vi "CRYSet Acquisition Editor Front Panel.vi"(11 "Vi Ref":refnum<vi>) -> ()   [LabVIEW 2013]
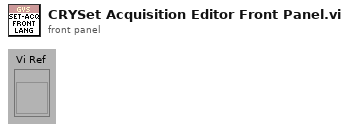
[diagram p1: front panel]
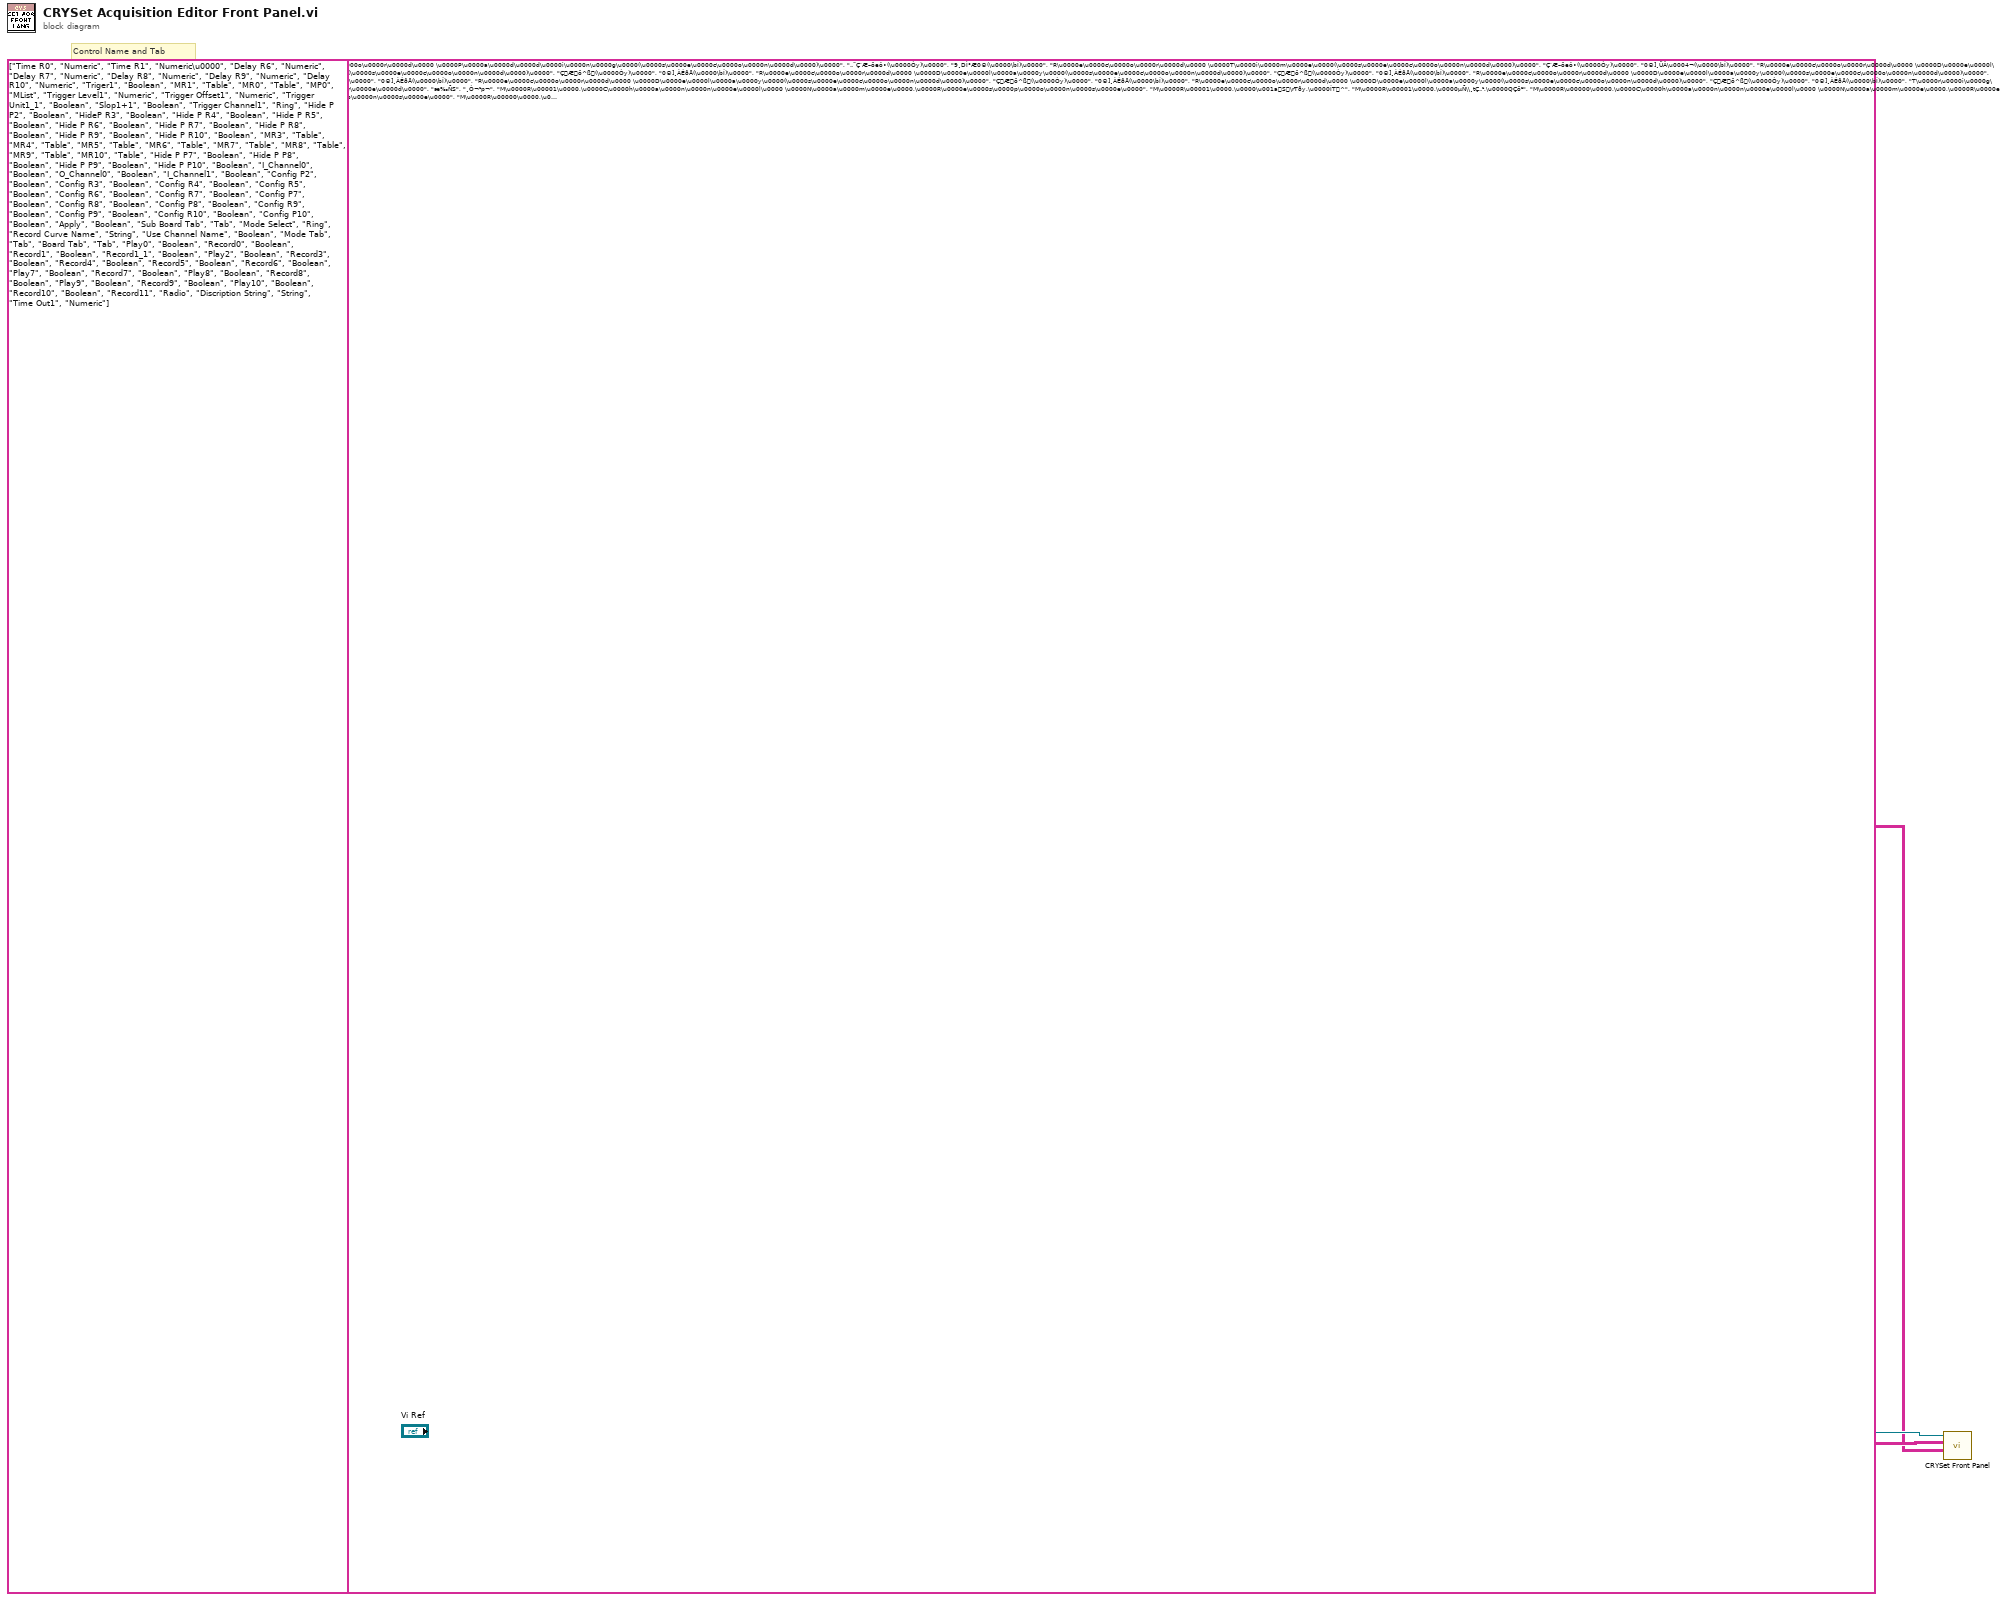
[diagram p0: block diagram]
diagram:
  # ","
  # "Caption, Tab Page, Multilist Header, Button 4"
  # "Control Type"
  # "Control Name and Tab"
  n1 = call "CRYSet Front Panel.vi"("Caption(Boolean Text)"=string[][] [["R\u0000e\u0000c\u0000o\u0000r\u0000d\u0000 \u0000P\u0000a\u0000d\u0000d\u0000i\u0000n\u0000g\u0000(\u0000s\u0000e\u0000c\u0000o\u0000n\u0000d\u0000)\u0000", "„˜Ç‘Æ–öeô•(\u0000Òy)\u0000", "9¸DÌ°Æ0®(\u0000\bÍ)\u0000"], ["R\u0000e\u0000c\u0000o\u0000r\u0000d\u0000 \u0000T\u0000i\u0000m\u0000e\u0000(\u0000s\u0000e\u0000c\u0000o\u0000n\u0000d\u0000)\u0000", "Ç‘Æ–öeô•(\u0000Òy)\u0000", "0®]¸ÜÂ\u0004¬(\u0000\bÍ)\u0000"], ["R\u0000e\u0000c\u0000o\u0000r\u0000d\u0000 \u0000D\u0000e\u0000l\u0000a\u0000y\u0000(\u0000s\u0000e\u0000c\u0000o\u0000n\u0000d\u0000)\u0000", "ÇÆö^ß(\u0000Òy)\u0000", "0®]¸ÀÉðÅ(\u0000\bÍ)\u0000"], ["R\u0000e\u0000c\u0000o\u0000r\u0000d\u0000 \u0000D\u0000e\u0000l\u0000a\u0000y\u0000(\u0000s\u0000e\u0000c\u0000o\u0000n\u0000d\u0000)\u0000", "ÇÆö^ß(\u0000Òy)\u0000", "0®]¸ÀÉðÅ(\u0000\bÍ)\u0000"], ["R\u0000e\u0000c\u0000o\u0000r\u0000d\u0000 \u0000D\u0000e\u0000l\u0000a\u0000y\u0000(\u0000s\u0000e\u0000c\u0000o\u0000n\u0000d\u0000)\u0000", "ÇÆö^ß(\u0000Òy)\u0000", "0®]¸ÀÉðÅ(\u0000\bÍ)\u0000"], ["R\u0000e\u0000c\u0000o\u0000r\u0000d\u0000 \u0000D\u0000e\u0000l\u0000a\u0000y\u0000(\u0000s\u0000e\u0000c\u0000o\u0000n\u0000d\u0000)\u0000", "ÇÆö^ß(\u0000Òy)\u0000", "0®]¸ÀÉðÅ(\u0000\bÍ)\u0000"], ["R\u0000e\u0000c\u0000o\u0000r\u0000d\u0000 \u0000D\u0000e\u0000l\u0000a\u0000y\u0000(\u0000s\u0000e\u0000c\u0000o\u0000n\u0000d\u0000)\u0000", "ÇÆö^ß(\u0000Òy)\u0000", "0®]¸ÀÉðÅ(\u0000\bÍ)\u0000"], ["T\u0000r\u0000i\u0000g\u0000g\u0000e\u0000r\u0000e\u0000d\u0000", "æ‰ÑS", "¸Ò¬¹p¬"], ["M\u0000R\u00001\u0000,\u0000C\u0000h\u0000a\u0000n\u0000n\u0000e\u0000l\u0000 \u0000N\u0000a\u0000m\u0000e\u0000,\u0000R\u0000e\u0000s\u0000p\u0000o\u0000n\u0000s\u0000e\u0000", "M\u0000R\u00001\u0000,\u0000\u001aS\rTðy,\u0000ÍT^", "M\u0000R\u00001\u0000,\u0000µÑ\\¸tÇ„¹,\u0000QÇõ²"], ["M\u0000R\u00000\u0000,\u0000C\u0000h\u0000a\u0000n\u0000n\u0000e\u0000l\u0000 \u0000N\u0000a\u0000m\u0000e\u0000,\u0000R\u0000e\u0000s\u0000p\u0000o\u0000n\u0000s\u0000e\u0000", "M\u0000R\u00000\u0000,\u0000\u001aS\rTðy,\u0000ÍT^", "M\u0000R\u00000\u0000,\u0000µÑ\\¸tÇ„¹,\u0000QÇõ²"], ["M\u0000P\u00000\u0000,\u0000C\u0000h\u0000a\u0000n\u0000n\u0000e\u0000l\u0000 \u0000N\u0000a\u0000m\u0000e\u0000,\u0000S\u0000t\u0000i\u0000m\u0000u\u0000l\u0000u\u0000s\u0000", "M\u0000P\u00000\u0000,\u0000\u001aS\rTðy,\u0000Ào±R", "M\u0000P\u0000,\u0000µÑ\\¸tÇ¹,\u0000Çù­"], ["T\u0000r\u0000i\u0000g\u0000g\u0000e\u0000r\u0000 \u0000L\u0000e\u0000v\u0000e\u0000l\u0000", "æ‰ÑS5us^", "¸Ò¬¹p¬\u0000É\u0004Ç"], ["T\u0000r\u0000i\u0000g\u0000g\u0000e\u0000r\u0000 \u0000O\u0000f\u0000f\u0000s\u0000e\u0000t\u0000(\u0000s\u0000)\u0000", "æ‰ÑSOPûy(\u0000s\u0000)\u0000", "¸Ò¬¹p¬¸Ó\u0004Ç(\u0000\bÍ)\u0000"], ["T\u0000r\u0000i\u0000g\u0000g\u0000e\u0000r\u0000 \u0000U\u0000n\u0000i\u0000t\u0000", "æ‰ÑSUSMO", "¸Ò¬¹p¬è²\u0004Ç"], ["S\u0000l\u0000o\u0000p\u0000e\u0000", "œe‡s", "½¬¬ÀÄ³"], ["T\u0000r\u0000i\u0000g\u0000g\u0000e\u0000r\u0000 \u0000C\u0000h\u0000a\u0000n\u0000n\u0000e\u0000l\u0000", "æÑS\u001aS", "¸Ò¬¹p¬µÑ\\¸"], ["H\u0000i\u0000d\u0000e\u0000 \u0000P\u0000a\u0000n\u0000e\u0000l\u0000", "Ïbg", "=Ì8»(Â0®0®"], ["H\u0000i\u0000d\u0000e\u0000 \u0000P\u0000a\u0000n\u0000e\u0000l\u0000", "Ïbg", "=Ì8»(Â0®0®"], ["H\u0000i\u0000d\u0000e\u0000 \u0000P\u0000a\u0000n\u0000e\u0000l\u0000", "Ïbg", "=Ì8»(Â0®0®"], ["H\u0000i\u0000d\u0000e\u0000 \u0000P\u0000a\u0000n\u0000e\u0000l\u0000", "Ïbg", "=Ì8»(Â0®0®"], ["H\u0000i\u0000d\u0000e\u0000 \u0000P\u0000a\u0000n\u0000e\u0000l\u0000", "Ïbg", "=Ì8»(Â0®0®"], ["H\u0000i\u0000d\u0000e\u0000 \u0000P\u0000a\u0000n\u0000e\u0000l\u0000", "Ïbg", "=Ì8»(Â0®0®"], ["H\u0000i\u0000d\u0000e\u0000 \u0000P\u0000a\u0000n\u0000e\u0000l\u0000", "Ïbg", "=Ì8»(Â0®0®"], ["H\u0000i\u0000d\u0000e\u0000 \u0000P\u0000a\u0000n\u0000e\u0000l\u0000", "Ïbg", "=Ì8»(Â0®0®"], ["H\u0000i\u0000d\u0000e\u0000 \u0000P\u0000a\u0000n\u0000e\u0000l\u0000", "Ïbg", "=Ì8»(Â0®0®"], ["M\u0000R\u00003\u0000,\u0000C\u0000h\u0000a\u0000n\u0000n\u0000e\u0000l\u0000 \u0000N\u0000a\u0000m\u0000e\u0000,\u0000R\u0000e\u0000s\u0000p\u0000o\u0000n\u0000s\u0000e\u0000", "M\u0000R\u00003\u0000,\u0000\u001aS\rTðy,\u0000ÍT^", "M\u0000R\u0000,\u0000µÑ\\¸tÇ„¹,\u0000QÇõ²"], ["M\u0000R\u00004\u0000,\u0000C\u0000h\u0000a\u0000n\u0000n\u0000e\u0000l\u0000 \u0000N\u0000a\u0000m\u0000e\u0000,\u0000R\u0000e\u0000s\u0000p\u0000o\u0000n\u0000s\u0000e\u0000", "M\u0000R\u00004\u0000,\u0000\u001aS\rTðy,\u0000ÍT^", "M\u0000R\u0000,\u0000µÑ\\¸tÇ„¹,\u0000QÇõ²"], ["M\u0000R\u00005\u0000,\u0000C\u0000h\u0000a\u0000n\u0000n\u0000e\u0000l\u0000 \u0000N\u0000a\u0000m\u0000e\u0000,\u0000R\u0000e\u0000s\u0000p\u0000o\u0000n\u0000s\u0000e\u0000", "M\u0000R\u00005\u0000,\u0000\u001aS\rTðy,\u0000ÍT^", "M\u0000R\u0000,\u0000µÑ\\¸tÇ„¹,\u0000QÇõ²"], ["M\u0000R\u00006\u0000,\u0000C\u0000h\u0000a\u0000n\u0000n\u0000e\u0000l\u0000 \u0000N\u0000a\u0000m\u0000e\u0000,\u0000R\u0000e\u0000s\u0000p\u0000o\u0000n\u0000s\u0000e\u0000", "M\u0000R\u00006\u0000,\u0000\u001aS\rTðy,\u0000ÍT^", "M\u0000R\u0000,\u0000µÑ\\¸tÇ„¹,\u0000QÇõ²"], ["M\u0000R\u00007\u0000,\u0000C\u0000h\u0000a\u0000n\u0000n\u0000e\u0000l\u0000 \u0000N\u0000a\u0000m\u0000e\u0000,\u0000R\u0000e\u0000s\u0000p\u0000o\u0000n\u0000s\u0000e\u0000", "M\u0000R\u00007\u0000,\u0000\u001aS\rTðy,\u0000ÍT^", "M\u0000R\u0000,\u0000µÑ\\¸tÇ„¹,\u0000QÇõ²"], ["M\u0000R\u00008\u0000,\u0000C\u0000h\u0000a\u0000n\u0000n\u0000e\u0000l\u0000 \u0000N\u0000a\u0000m\u0000e\u0000,\u0000R\u0000e\u0000s\u0000p\u0000o\u0000n\u0000s\u0000e\u0000", "M\u0000R\u00008\u0000,\u0000\u001aS\rTðy,\u0000ÍT^", "M\u0000R\u0000,\u0000µÑ\\¸tÇ„¹,\u0000QÇõ²"], ["M\u0000R\u00009\u0000,\u0000C\u0000h\u0000a\u0000n\u0000n\u0000e\u0000l\u0000 \u0000N\u0000a\u0000m\u0000e\u0000,\u0000R\u0000e\u0000s\u0000p\u0000o\u0000n\u0000s\u0000e\u0000", "M\u0000R\u00009\u0000,\u0000\u001aS\rTðy,\u0000ÍT^", "M\u0000R\u0000,\u0000µÑ\\¸tÇ„¹,\u0000QÇõ²"], ["M\u0000R\u00001\u00000\u0000,\u0000C\u0000h\u0000a\u0000n\u0000n\u0000e\u0000l\u0000 \u0000N\u0000a\u0000m\u0000e\u0000,\u0000R\u0000e\u0000s\u0000p\u0000o\u0000n\u0000s\u0000e\u0000", "M\u0000R\u00001\u00000\u0000,\u0000\u001aS\rTðy,\u0000ÍT^", "M\u0000R\u0000,\u0000µÑ\\¸tÇ„¹,\u0000QÇõ²"], ["H\u0000i\u0000d\u0000e\u0000 \u0000P\u0000a\u0000n\u0000e\u0000l\u0000", "Ïbg", "=Ì8»(Â0®0®"], ["H\u0000i\u0000d\u0000e\u0000 \u0000P\u0000a\u0000n\u0000e\u0000l\u0000", "Ïbg", "=Ì8»(Â0®0®"], ["H\u0000i\u0000d\u0000e\u0000 \u0000P\u0000a\u0000n\u0000e\u0000l\u0000", "Ïbg", "=Ì8»(Â0®0®"], ["H\u0000i\u0000d\u0000e\u0000 \u0000P\u0000a\u0000n\u0000e\u0000l\u0000", "Ïbg", "=Ì8»(Â0®0®"], ["I\u0000n\u0000p\u0000u\u0000t\u0000 \u0000C\u0000h\u0000a\u0000n\u0000n\u0000e\u0000l\u0000", "eQ\u001aS", "…Çl­µÑ\\¸"], ["O\u0000u\u0000t\u0000p\u0000u\u0000t\u0000 \u0000C\u0000h\u0000a\u0000n\u0000n\u0000e\u0000l\u0000", "úQ\u001aS", "œÍl­µÑ\\¸"], ["I\u0000n\u0000p\u0000u\u0000t\u0000 \u0000C\u0000h\u0000a\u0000n\u0000n\u0000e\u0000l\u0000", "eQ\u001aS", "…Çl­µÑ\\¸"], ["C\u0000o\u0000n\u0000f\u0000i\u0000g\u0000u\u0000r\u0000e\u0000 \u0000G\u0000e\u0000n\u0000e\u0000r\u0000a\u0000t\u0000o\u0000r\u0000", "M‘nÑS\u001fuhV", "\u001c¼ÝÀ0®l­1Á"], ["C\u0000o\u0000n\u0000f\u0000i\u0000g\u0000u\u0000r\u0000e\u0000 \u0000R\u0000e\u0000c\u0000o\u0000r\u0000d\u0000", "M‘n°‹U_", "0®]¸l­1Á"], ["C\u0000o\u0000n\u0000f\u0000i\u0000g\u0000u\u0000r\u0000e\u0000 \u0000R\u0000e\u0000c\u0000o\u0000r\u0000d\u0000", "M‘n°‹U_", "0®]¸l­1Á"], ["C\u0000o\u0000n\u0000f\u0000i\u0000g\u0000u\u0000r\u0000e\u0000 \u0000R\u0000e\u0000c\u0000o\u0000r\u0000d\u0000", "M‘n°‹U_", "0®]¸l­1Á"], ["C\u0000o\u0000n\u0000f\u0000i\u0000g\u0000u\u0000r\u0000e\u0000 \u0000R\u0000e\u0000c\u0000o\u0000r\u0000d\u0000", "M‘n°‹U_", "0®]¸l­1Á"], ["C\u0000o\u0000n\u0000f\u0000i\u0000g\u0000u\u0000r\u0000e\u0000 \u0000R\u0000e\u0000c\u0000o\u0000r\u0000d\u0000", "M‘n°‹U_", "0®]¸l­1Á"], ["C\u0000o\u0000n\u0000f\u0000i\u0000g\u0000u\u0000r\u0000e\u0000 \u0000G\u0000e\u0000n\u0000e\u0000r\u0000a\u0000t\u0000o\u0000r\u0000", "M‘nÑS\u001fuhV", "\u001c¼ÝÀ0®l­1Á"], ["C\u0000o\u0000n\u0000f\u0000i\u0000g\u0000u\u0000r\u0000e\u0000 \u0000R\u0000e\u0000c\u0000o\u0000r\u0000d\u0000", "M‘n°‹U_", "0®]¸l­1Á"], ["C\u0000o\u0000n\u0000f\u0000i\u0000g\u0000u\u0000r\u0000e\u0000 \u0000G\u0000e\u0000n\u0000e\u0000r\u0000a\u0000t\u0000o\u0000r\u0000", "M‘nÑS\u001fuhV", "\u001c¼ÝÀ0®l­1Á"], ["C\u0000o\u0000n\u0000f\u0000i\u0000g\u0000u\u0000r\u0000e\u0000 \u0000R\u0000e\u0000c\u0000o\u0000r\u0000d\u0000", "M‘n°‹U_", "0®]¸l­1Á"], ["C\u0000o\u0000n\u0000f\u0000i\u0000g\u0000u\u0000r\u0000e\u0000 \u0000G\u0000e\u0000n\u0000e\u0000r\u0000a\u0000t\u0000o\u0000r\u0000", "M‘nÑS\u001fuhV", "\u001c¼ÝÀ0®l­1Á"], ["C\u0000o\u0000n\u0000f\u0000i\u0000g\u0000u\u0000r\u0000e\u0000 \u0000R\u0000e\u0000c\u0000o\u0000r\u0000d\u0000", "M‘n°‹U_", "0®]¸l­1Á"], ["C\u0000o\u0000n\u0000f\u0000i\u0000g\u0000u\u0000r\u0000e\u0000 \u0000G\u0000e\u0000n\u0000e\u0000r\u0000a\u0000t\u0000o\u0000r\u0000", "M‘nÑS\u001fuhV", "\u001c¼ÝÀ0®l­1Á"], ["A\u0000p\u0000p\u0000l\u0000y\u0000,\u0000S\u0000t\u0000o\u0000p\u0000", "”^(u,\u0000\\Pbk", "\u0001È©Æ,\u0000\u0015ÈÀÉ"], ["S\u0000e\u0000t\u0000t\u0000i\u0000n\u0000g\u0000,\u0000H\u0000e\u0000l\u0000p\u0000", "¾‹n,\u0000.^©R", "$Á\u0015È,\u0000Ä³ÀÆÐ¹"], ["M\u0000o\u0000d\u0000e\u0000 \u0000S\u0000e\u0000l\u0000e\u0000c\u0000t\u0000,\u0000P\u0000l\u0000a\u0000y\u0000 \u0000&\u0000 \u0000R\u0000e\u0000c\u0000o\u0000r\u0000d\u0000,\u0000R\u0000e\u0000c\u0000o\u0000r\u0000d\u0000,\u0000S\u0000i\u0000g\u0000n\u0000a\u0000l\u0000 \u0000G\u0000e\u0000n\u0000e\u0000r\u0000a\u0000t\u0000o\u0000r\u0000,\u0000M\u0000u\u0000l\u0000t\u0000i\u0000m\u0000e\u0000t\u0000e\u0000r\u0000,\u0000O\u0000s\u0000c\u0000i\u0000l\u0000l\u0000o\u0000s\u0000c\u0000o\u0000p\u0000e\u0000,\u0000S\u0000p\u0000e\u0000c\u0000t\u0000r\u0000u\u0000m\u0000 \u0000A\u0000n\u0000a\u0000l\u0000y\u0000z\u0000e\u0000r\u0000,\u0000R\u0000e\u0000a\u0000l\u0000 \u0000T\u0000i\u0000m\u0000e\u0000 \u0000A\u0000n\u0000a\u0000l\u0000y\u0000z\u0000e\u0000r\u0000,\u0000G\u0000e\u0000n\u0000e\u0000r\u0000a\u0000t\u0000o\u0000r\u0000 \u0000&\u0000 \u0000M\u0000u\u0000l\u0000t\u0000i\u0000m\u0000e\u0000t\u0000e\u0000r\u0000,\u0000G\u0000e\u0000n\u0000e\u0000r\u0000a\u0000t\u0000o\u0000r\u0000 \u0000&\u0000 \u0000O\u0000s\u0000c\u0000i\u0000l\u0000l\u0000o\u0000s\u0000c\u0000o\u0000p\u0000e\u0000,\u0000G\u0000e\u0000n\u0000e\u0000r\u0000a\u0000t\u0000o\u0000r\u0000 \u0000&\u0000 \u0000S\u0000p\u0000e\u0000c\u0000t\u0000r\u0000u\u0000m\u0000,\u0000G\u0000e\u0000n\u0000e\u0000r\u0000a\u0000t\u0000o\u0000r\u0000 \u0000&\u0000 \u0000R\u0000T\u0000A\u0000,\u0000R\u0000e\u0000a\u0000d\u0000 \u0000f\u0000r\u0000o\u0000m\u0000 \u0000D\u0000C\u0000 \u0000C\u0000o\u0000n\u0000n\u0000e\u0000c\u0000t\u0000", "!j\u000f_\téb,\u0000­d>eTÇÆ,\u0000ÇÆ,\u0000áO÷SÑS\u001fuhV,\u0000\u001aYRýh,\u0000:yâlhV,\u00001\u0006RgêN,\u0000[öe1\u0006RgêN,\u0000áO÷SÑS\u001fuhV/\u0000\u001aYRýh,\u0000áO÷SÑS\u001fuhV/\u0000:yâlhV,\u0000áO÷SÑS\u001fuhV/\u00001\u0006RgêN,\u0000áO÷SÑS\u001fuhV/\u0000[öe1\u0006RgêN,\u0000ûÖSôvAmÞ¥c", ")¼ÝÂ ÁÝÐ,\u0000¬ÇÝÀü¬ \u00000®]¸,\u00000®]¸,\u0000àÂ8Ö\u001c¼ÝÀ0®,\u0000Ì¹¥²!Î\u0015ÈÄ¬0®,\u0000$Æ0Å\\¸¤ÂTÏ\u0004Õ,\u0000¤Â™Ó¸Òt¹„½\u001dÁ0®,\u0000%ÆÀÐ\f¾„½\u001dÁ0®,\u0000àÂ8Ö\u001c¼ÝÀ0®@Æ \u0000Ì¹¥²!Î\u0015ÈÄ¬0®,\u0000àÂ8Ö\u001c¼ÝÀ0®@Æ \u0000$Æ0Å\\¸¤ÂTÏ\u0004Õ,\u0000àÂ8Ö\u001c¼ÝÀ0®@Æ \u0000¤Â™Ó¸Òt¹„½\u001dÁ0®,\u0000àÂ8Ö\u001c¼ÝÀ0®@Æ \u0000%ÆÀÐ\f¾„½\u001dÁ0®,\u0000ÁÉX¹(¸°¬0®\\¸ \u0000€½0Ñ \u0000}Ç0®"], ["R\u0000e\u0000c\u0000o\u0000r\u0000d\u0000 \u0000C\u0000u\u0000r\u0000v\u0000e\u0000 \u0000N\u0000a\u0000m\u0000e\u0000", "°‹U_òf¿~\rTðy", "0®]¸á¬ ÁtÇ„¹"], ["U\u0000s\u0000e\u0000 \u0000C\u0000h\u0000a\u0000n\u0000n\u0000e\u0000l\u0000 \u0000N\u0000a\u0000m\u0000e\u0000", "O(u\u001aS\rTðy", "µÑ\\¸tÇ„¹¬¹©Æ"], ["M\u0000o\u0000d\u0000e\u0000 \u0000T\u0000a\u0000b\u0000", "M\u0000o\u0000d\u0000e\u0000 \u0000T\u0000a\u0000b\u0000", "M\u0000o\u0000d\u0000e\u0000 \u0000T\u0000a\u0000b\u0000c\u0000"], ["B\u0000o\u0000a\u0000r\u0000d\u0000 \u0000T\u0000a\u0000b\u0000", "B\u0000o\u0000a\u0000r\u0000d\u0000 \u0000T\u0000a\u0000b\u0000", "B\u0000o\u0000a\u0000r\u0000d\u0000 \u0000T\u0000a\u0000b\u0000"], ["P\u0000l\u0000a\u0000y\u0000", "­d>e", "¬ÇÝÀ"], ["R\u0000e\u0000c\u0000o\u0000r\u0000d\u0000", "ǑƖ", "0®]¸"], ["R\u0000e\u0000c\u0000o\u0000r\u0000d\u0000", "ǑƖ", "0®]¸"], ["R\u0000e\u0000c\u0000o\u0000r\u0000d\u0000 \u0000T\u0000r\u0000i\u0000g\u0000g\u0000e\u0000r\u0000", "Ç‘Æ–æ‰ÑS", "0®]¸¸Ò¬¹p¬"], ["P\u0000l\u0000a\u0000y\u0000", "­d>e", "¬ÇÝÀ"], ["R\u0000e\u0000c\u0000o\u0000r\u0000d\u0000", "ǑƖ", "0®]¸"], ["R\u0000e\u0000c\u0000o\u0000r\u0000d\u0000", "ǑƖ", "0®]¸"], ["R\u0000e\u0000c\u0000o\u0000r\u0000d\u0000", "ǑƖ", "0®]¸"], ["R\u0000e\u0000c\u0000o\u0000r\u0000d\u0000", "ǑƖ", "0®]¸"], ["P\u0000l\u0000a\u0000y\u0000", "­d>e", "¬ÇÝÀ"], ["R\u0000e\u0000c\u0000o\u0000r\u0000d\u0000", "ǑƖ", "0®]¸"], ["P\u0000l\u0000a\u0000y\u0000", "­d>e", "¬ÇÝÀ"], ["R\u0000e\u0000c\u0000o\u0000r\u0000d\u0000", "ǑƖ", "0®]¸"], ["P\u0000l\u0000a\u0000y\u0000", "­d>e", "¬ÇÝÀ"], ["R\u0000e\u0000c\u0000o\u0000r\u0000d\u0000", "ǑƖ", "0®]¸"], ["P\u0000l\u0000a\u0000y\u0000", "­d>e", "¬ÇÝÀ"], ["R\u0000e\u0000c\u0000o\u0000r\u0000d\u0000", "ǑƖ", "0®]¸"], ["R\u0000e\u0000c\u0000o\u0000r\u0000d\u0000,\u0000A\u0000 \u0000(\u0000i\u0000n\u0000 \u0000V\u0000o\u0000l\u0000t\u0000a\u0000g\u0000e\u0000 \u0000S\u0000o\u0000u\u0000r\u0000c\u0000e\u0000 \u0000M\u0000o\u0000d\u0000e\u0000)\u0000,\u0000V\u0000 \u0000(\u0000i\u0000n\u0000 \u0000C\u0000u\u0000r\u0000r\u0000e\u0000n\u0000t\u0000 \u0000S\u0000o\u0000u\u0000r\u0000c\u0000e\u0000 \u0000M\u0000o\u0000d\u0000e\u0000)\u0000", "ÇÆ,\u0000A\u0000(\u00005uSn!j\u000f_)\u0000,\u0000V\u0000(\u00005uAmn!j\u000f_)\u0000", "0®]¸,\u0000TÅ˜ÓDÅ(\u0000\u0004ÈUÅÐÆœÌ)¼ÝÂÐÅ\u001cÁ)\u0000,\u0000ü¼¸Ò(\u0000\u0004ÈX¹ÐÆœÌ)¼ÝÂÐÅ\u001cÁ)\u0000"], ["D\u0000i\u0000s\u0000c\u0000r\u0000i\u0000p\u0000t\u0000i\u0000o\u0000n\u0000 \u0000S\u0000t\u0000r\u0000i\u0000n\u0000g\u0000,\u0000F\u0000u\u0000n\u0000c\u0000t\u0000i\u0000o\u0000n\u0000 \u0000d\u0000e\u0000s\u0000c\u0000r\u0000i\u0000p\u0000t\u0000i\u0000o\u0000n\u0000:\u0000 \u0000v\u0000i\u0000a\u0000 \u0000U\u0000S\u0000B\u0000,\u0000 \u0000a\u0000 \u0000s\u0000i\u0000n\u0000g\u0000l\u0000e\u0000 \u0000m\u0000e\u0000a\u0000s\u0000u\u0000r\u0000e\u0000d\u0000 \u0000v\u0000a\u0000l\u0000u\u0000e\u0000 \u0000i\u0000s\u0000 \u0000r\u0000e\u0000a\u0000d\u0000 \u0000f\u0000r\u0000o\u0000m\u0000 \u0000t\u0000h\u0000e\u0000 \u0000a\u0000s\u0000s\u0000i\u0000g\u0000n\u0000e\u0000d\u0000 \u0000D\u0000C\u0000 \u0000c\u0000o\u0000n\u0000n\u0000e\u0000c\u0000t\u0000 \u0000d\u0000e\u0000v\u0000i\u0000c\u0000e\u0000.\u0000", "ÏcðW[&{2N,\u0000RýÏcð:\u0000\u001aÇU\u0000S\u0000B\u0000¥cãS,\u0000\u0000N*NUS\u0000NvKmÏ<P/fÎN\u0007c[vôvAmÞ¥c¾\u0007YûÖS.\u0000", "8»Ç,¸,\u00000®¥²\u001cÁ Â:\u0000U\u0000S\u0000B\u0000|¹ \u0000µÑtÕ\u001cÁ \u0000!Î\u0015È\u001c´ \u0000è²\u001cÂ\u0012¬@Ç \u0000`Õù²\u001c´ \u0000ÁÉX¹(¸°¬¥ÇXÎ\\¸½0Ñ \u0000}Ç²ä².\u0000"], ["T\u0000i\u0000m\u0000e\u0000 \u0000O\u0000u\u0000t\u0000(\u0000s\u0000)\u0000", "öeô•Ó~_g(\u0000s\u0000)\u0000", "DÆÌ¸ÜÂ\u0004¬"]], "Control ID and Type(Label Name, Type)"=string[][] [["Time R0", "Numeric"], ["Time R1", "Numeric\u0000"], ["Delay R6", "Numeric"], ["Delay R7", "Numeric"], ["Delay R8", "Numeric"], ["Delay R9", "Numeric"], ["Delay R10", "Numeric"], ["Triger1", "Boolean"], ["MR1", "Table"], ["MR0", "Table"], ["MP0", "MList"], ["Trigger Level1", "Numeric"], ["Trigger Offset1", "Numeric"], ["Trigger Unit1_1", "Boolean"], ["Slop1+1", "Boolean"], ["Trigger Channel1", "Ring"], ["Hide P P2", "Boolean"], ["HideP R3", "Boolean"], ["Hide P R4", "Boolean"], ["Hide P R5", "Boolean"], ["Hide P R6", "Boolean"], ["Hide P R7", "Boolean"], ["Hide P R8", "Boolean"], ["Hide P R9", "Boolean"], ["Hide P R10", "Boolean"], ["MR3", "Table"], ["MR4", "Table"], ["MR5", "Table"], ["MR6", "Table"], ["MR7", "Table"], ["MR8", "Table"], ["MR9", "Table"], ["MR10", "Table"], ["Hide P P7", "Boolean"], ["Hide P P8", "Boolean"], ["Hide P P9", "Boolean"], ["Hide P P10", "Boolean"], ["I_Channel0", "Boolean"], ["O_Channel0", "Boolean"], ["I_Channel1", "Boolean"], ["Config P2", "Boolean"], ["Config R3", "Boolean"], ["Config R4", "Boolean"], ["Config R5", "Boolean"], ["Config R6", "Boolean"], ["Config R7", "Boolean"], ["Config P7", "Boolean"], ["Config R8", "Boolean"], ["Config P8", "Boolean"], ["Config R9", "Boolean"], ["Config P9", "Boolean"], ["Config R10", "Boolean"], ["Config P10", "Boolean"], ["Apply", "Boolean"], ["Sub Board Tab", "Tab"], ["Mode Select", "Ring"], ["Record Curve Name", "String"], ["Use Channel Name", "Boolean"], ["Mode Tab", "Tab"], ["Board Tab", "Tab"], ["Play0", "Boolean"], ["Record0", "Boolean"], ["Record1", "Boolean"], ["Record1_1", "Boolean"], ["Play2", "Boolean"], ["Record3", "Boolean"], ["Record4", "Boolean"], ["Record5", "Boolean"], ["Record6", "Boolean"], ["Play7", "Boolean"], ["Record7", "Boolean"], ["Play8", "Boolean"], ["Record8", "Boolean"], ["Play9", "Boolean"], ["Record9", "Boolean"], ["Play10", "Boolean"], ["Record10", "Boolean"], ["Record11", "Radio"], ["Discription String", "String"], ["Time Out1", "Numeric"]], "Vi Ref"="Vi Ref") -> ()  [unwired: 9 in]
